vi "Read SSH User Directory.vi"(8 "error in (no error)":errorcluster, 11 "OpenSSH Client in":refnum<class "OpenSSH Client.lvclass">) -> (0 "error out":errorcluster, 2 "Path":path, 3 "OpenSSH Client out":refnum<class "OpenSSH Client.lvclass">)   [LabVIEW 2020, in "NI_SSH.lvlib" / "OpenSSH Client.lvclass"]
uses:
  <vilib>/net/SSH/Client/OpenSSH/OpenSSH Client.lvclass
  <vilib>/Utility/sysdir.llb/System Directory Type.ctl
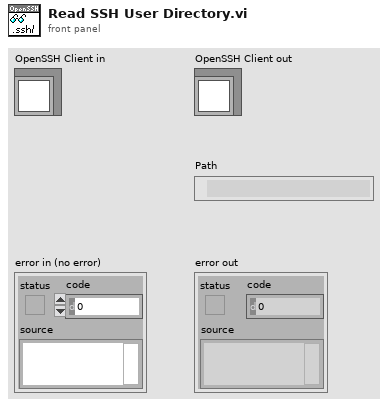
[diagram p1: front panel]
types:
  T1 = typedef "System Directory Type.ctl" = i32
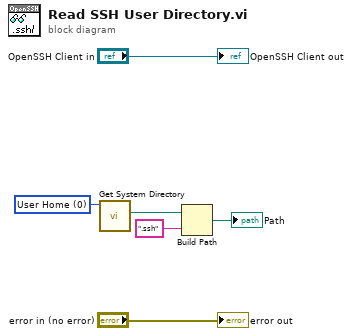
[diagram p0: block diagram]
diagram:
  w5 = T1 0 items=["User Home"=0, "User Desktop"=1, "User Documents"=2, "User Application Data"=3, "User Preferences"=4, "User Temporary"=5, "Public Documents"=6, "Public Application Data"=7, "Public Preferences"=8, "Public Cache"=13, "System Core Libraries"=9, "System Installed Libraries"=10, "Application Files"=11, "Boot Volume Root"=12] ("system directory type")
  n1 = call <vilib>:"Get System Directory.vi"("system directory type"=w5) -> ("system directory"=w4:path)  [unwired: 10 in]
  n2 = Build Path(base path=w4, name or relative path=".ssh") -> (appended path=→"Path":path)
  "error out" <- "error in (no error)"
  "OpenSSH Client out" <- "OpenSSH Client in"
